vi "蠕动泵状态读取.vi"(8 "error in (no error)":errorcluster, 11 "Slave ID":T1) -> (0 "error out":errorcluster, 2 "脉冲数":i32, 3 "频率":i32)   [LabVIEW 2016, in "质控单元V1.lvlib"]
uses:
  <vilib>/Plasmionique/MB Master/MB_Master/MB_Master.lvclass
  <vilib>/Plasmionique/MB Master/MB Master.lvlib
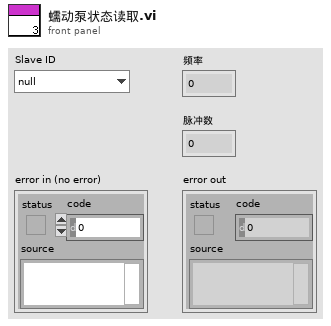
[diagram p1: front panel]
types:
  T1 = typedef "质控单元V1.lvlib/质控slave id.ctl" = enum16{"null", "氨氮", "总磷", "CODMn", "CODCr", "总氮"}
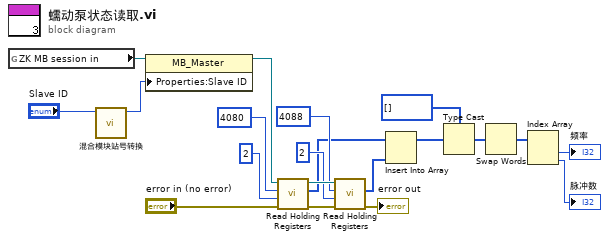
[diagram p0: block diagram]
diagram:
  n1 = global read "ZK非断电保存全局变量.vi" "ZK MB session in"() -> (w19:refnum<class "MB_Master.lvclass">)
  n2 = call "混合模块站号转换.vi"("Slave ID输入"="Slave ID") -> ("Slave ID输出"=w15:T1)  [unwired: 10 in]
  n3 = property class="MB_Master"(reference=w19, "Properties:Slave ID"=w15) -> (reference out=w18:refnum<class "MB_Master.lvclass">)  [unwired: 1 in, 1 out]
  n4 = call <vilib>:"Read Holding Registers.vi"("error in (no error)"="error in (no error)", "quantity"=u16 2, "starting address"=u16 4080, "MB session in"=w18) -> ("error out"=w13:errorcluster, "Registers"=w8:u16[], "MB session out"=w11:refnum<class "MB_Master.lvclass">)  [unwired: 5 in]
  n5 = call <vilib>:"Read Holding Registers.vi"("error in (no error)"=w13, "quantity"=u16 2, "starting address"=u16 4088, "MB session in"=w11) -> ("error out"=→"error out":errorcluster, "Registers"=w7:u16[])  [unwired: 5 in, 1 out]
  n6 = Insert Into Array(array=w8, new element=w7) -> (w6:u16[])  [unwired: 1 in]
  n7 = Type Cast(type=i32[] [], x=w6) -> (*(type *) &x=w4:i32[])
  n8 = Swap Words(1:w4) -> (0:w1:i32[])
  n9 = Index Array(array=w1) -> (element #1=→"频率":i32, element #2=→"脉冲数":i32)  [unwired: 2 in]
